vi "Move To Home.vi"(7 "Move if Same":bool=TRUE, 8 "error in":errorcluster, 9 "Speed(mm/s)":dbl=50.0, 11 "Gantry in":refnum<class "Gantry Class.lvclass">) -> (0 "error out":errorcluster, 3 "Gantry out":refnum<class "Gantry Class.lvclass">)   [LabVIEW 2011, in "Gantry Class.lvclass"]
uses:
  Gantry Class.lvclass
  Config Manager Class/Type Definitions/Named Position.ctl
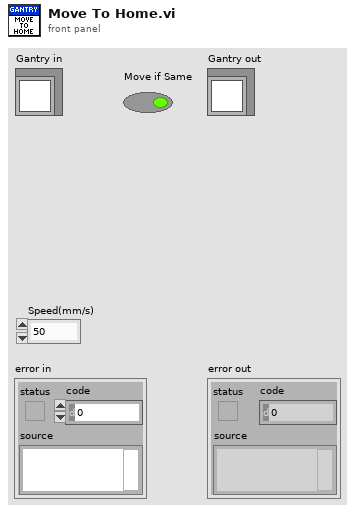
[diagram p1: front panel]
types:
  T1 = typedef "Named Position.ctl" = enum16{"home", "module_chuck_0", "module_chuck_1", "module_chuck_2", "module_chuck_3", "module_chuck_4", "glue_reservoir_chuck", "stamp_tool_chuck", "weight_tool_chuck", "needle_calibration", "tool_rack_pos_0_in", "tool_rack_pos_0_out", "tool_rack_pos_1_in", "tool_rack_pos_1_out", "tool_rack_pos_2_in", "tool_rack_pos_2_out", "front_load_position"}
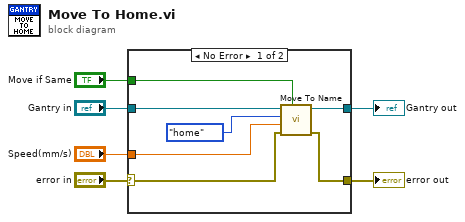
[diagram p0: block diagram]
diagram:
  n1 = case shown="No Error" "error in" {
    selector: "error in" -> [w9 w15]
    tunnel: [w8 w15] -> w2
    tunnel: [w10 w14] -> w1
    tunnel: "Gantry in" -> [w13 w14]
    tunnel: "Move if Same" -> [w12 _]
    tunnel: "Speed(mm/s)" -> [w11 _]
    frame No Error {
      n2 = call-dynamic "Move To Name.vi"("Move if Same"=w12, "error in"=w9, "Speed(mm/s)"=w11, "Destination"=Named_Position."home", "Gantry in"=w13) -> ("error out"=w8:errorcluster, "Gantry out"=w10:refnum<class "Gantry Class.lvclass">)  [unwired: 5 in]
    }
    frame Error {
    }
  }
  "error out" <- w2
  "Gantry out" <- w1
